vi "trash_Remove FIFO Instance.vi"(8 "error in (no error)":errorcluster, 10 "Publisher to Remove":string, 11 "Publisher Array in":refnum<class "CIFChannels.lvclass">[](array[class])) -> (0 "error out":errorcluster, 3 "Publisher Array out":refnum<class "CIFChannels.lvclass">[](array[class]))   [LabVIEW 2021]
uses:
  CIFChannels/CIFChannels.lvclass
  ChannelCommon.lvlib
  typedef/Errors.ctl
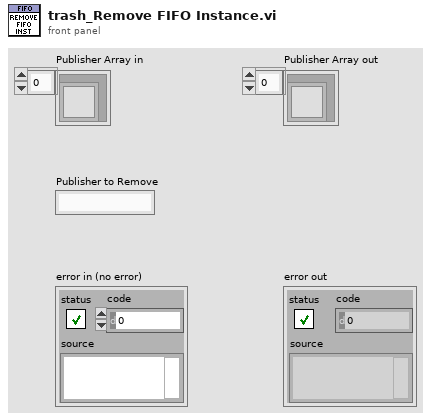
[diagram p1: front panel]
types:
  T1 = typedef "ChannelCommon.lvlib/Errors.ctl" = enum16{"gRPC Server Not Found", "Duplicate Channel", "Missing Channel", "Incorrect Type", "Flatten Error", "Unflatten Data", "Channel Length", "Plugin Connection", "gRPC Server Connection", "FIFO Unflatten", "Required Override", "Remove Not Found"}
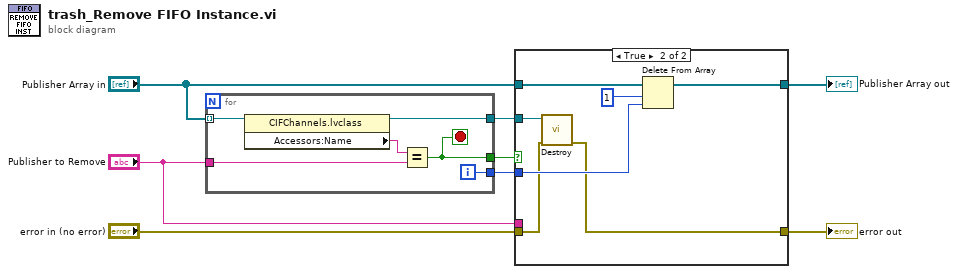
[diagram p0: block diagram]
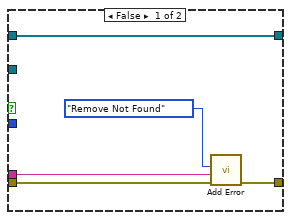
[diagram p2: hidden frame]
diagram:
  n1 = for {
    tunnel: "Publisher Array in" -> [w14] mode=indexing
    tunnel: "Publisher to Remove" -> [w12]
    tunnel: [w11] -> w8
    tunnel: [w10] -> w7
    tunnel: [w9] -> w6
    i -> [w9]
    stop <- w10 stop-if-true
    n2 = property class="CIFChannels.lvclass"(reference=w14) -> (reference out=w11:refnum<class "CIFChannels.lvclass">, "Accessors:Name"=w13:string)  [unwired: 1 in, 1 out]
    n3 = Equal?(x=w13, y=w12) -> (x = y?=w10:bool)
  }
  n4 = case shown="True" w7 {
    tunnel: "Publisher Array in" -> [w19 w26]
    tunnel: w8 -> [_ w25]
    tunnel: w6 -> [_ w24]
    tunnel: "error in (no error)" -> [w18 w22]
    tunnel: [w17 w21] -> w2
    tunnel: [w19 w20] -> w4
    tunnel: "Publisher to Remove" -> [w15 _]
    frame False {
      n5 = call "Add Error.vi"("error in (no error)"=w18, "String to Append"=w15, "Error"=Errors."Remove Not Found") -> ("error out"=w17:errorcluster)  [unwired: 8 in]
    }
    frame True {
      n6 = call-dynamic "Destroy.vi"("error in (no error)"=w22, "CIFChannels in"=w25) -> ("error out"=w21:errorcluster)  [unwired: 8 in, 1 out]
      n7 = Delete From Array(array=w26, length=1, index=w24) -> (array with subset deleted=w20:refnum<class "CIFChannels.lvclass">[])  [unwired: 1 out]
    }
  }
  "Publisher Array out" <- w4
  "error out" <- w2
